vi "Begin.vi"(11 "Image Size":T1=enum."160x120") -> (0 "error out":errorcluster)   [LabVIEW 2013]
doc: "Called before other user functions, this VI is expected to open initial I/O refnums, load in file data, and do all program initialization. Notice that the <B>error out</B> terminal is simply used for data flow. Wiring it to other structures or subVIs ensures that this VI runs first."
uses:
  <vilib>/Rock Robotics/WPI/Camera/WPI_CameraImageSize.ctl
  <vilib>/Rock Robotics/SystemInterfaces/DIO/FPGA_DIOPWMChannel.ctl
  <vilib>/Rock Robotics/WPI/Solenoid/WPI_SolenoidChannel.ctl
  <vilib>/Rock Robotics/SystemInterfaces/Typedef/FPGA_TypedefDigitalModule.ctl
  <vilib>/Rock Robotics/SystemInterfaces/DIO/FPGA_DIOChannel.ctl
  <vilib>/Rock Robotics/SystemInterfaces/DIO/FPGA_DIORelayChannel.ctl
  <vilib>/Rock Robotics/WPI/DriverStation/WPI_DriverStationRobotMode2.ctl
  <vilib>/Rock Robotics/WPI/Joystick/WPI_JoystickDeviceEnum.ctl
  <vilib>/Rock Robotics/WPI/MotorControl/WPI_MotorControlOpen Talon.vi
  <vilib>/Rock Robotics/WPI/Solenoid/WPI_SolenoidOpenSingle.vi
  <vilib>/Rock Robotics/WPI/Compressor/WPI_CompressorGetSetRefNum.vi
  Robot Global Data.vi
  <vilib>/Rock Robotics/WPI/Camera/WPI_CameraWhite Balance Values.ctl
  <vilib>/Rock Robotics/WPI/Camera/WPI_CameraExposure Values.ctl
  <vilib>/Rock Robotics/WPI/Camera/WPI_CameraFrameRate.ctl
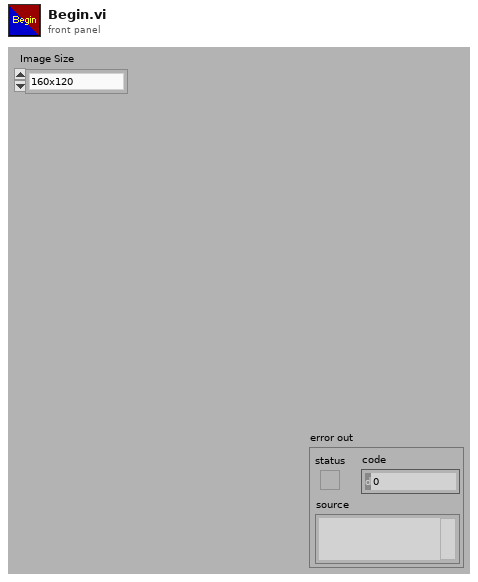
[diagram p1: front panel]
types:
  T1 = typedef "WPI_CameraImageSize.ctl" = enum16{"640x480", "320x240", "160x120"}
  T2 = typedef "FPGA_DIOPWMChannel.ctl" = enum8{"PWM 1", "PWM 2", "PWM 3", "PWM 4", "PWM 5", "PWM 6", "PWM 7", "PWM 8", "PWM 9", "PWM 10", "Invalid"}
  T3 = typedef "WPI_SolenoidChannel.ctl" = enum8{"Solenoid 1", "Solenoid 2", "Solenoid 3", "Solenoid 4", "Solenoid 5", "Solenoid 6", "Solenoid 7", "Solenoid 8", "Invalid"}
  T4 = typedef "FPGA_DIORelayChannel.ctl" = enum8{"Relay 1", "Relay 2", "Relay 3", "Relay 4", "Relay 5", "Relay 6", "Relay 7", "Relay 8", "Invalid"}
  T5 = typedef "FPGA_DIOChannel.ctl" = enum8{"DIO 1", "DIO 2", "DIO 3", "DIO 4", "DIO 5", "DIO 6", "DIO 7", "DIO 8", "DIO 9", "DIO 10", "DIO 11", "DIO 12", "DIO 13", "DIO 14", "Invalid"}
  T6 = typedef "WPI_JoystickDeviceEnum.ctl" = enum16{"USB 1", "USB 2", "USB 3", "USB 4", "Kinect 1", "Kinect 2"}
  T7 = typedef "WPI_DriverStationRobotMode2.ctl" = enum16{"Autonomous Disabled", "Autonomous Enabled", "Teleop Disabled", "Teleop Enabled", "Timeout", "Finish", "Test Disabled", "Test Enabled"}
  T8 = typedef "WPI_CameraFrameRate.ctl" = u32
  T9 = typedef "WPI_CameraExposure Values.ctl" = enum16{"Auto", "Flicker-free 50 Hz", "Flicker-free 60 Hz", "Hold current"}
  T10 = typedef "WPI_CameraWhite Balance Values.ctl" = enum16{"Auto", "Fixed indoor", "Fixed outdoor 1", "Fixed outdoor 2", "Fixed fluorescent 1", "Fixed fluorescent 2", "Hold current"}
  T11 = typedef "WPI_MotorControlDeviceRef.ctl" = cluster{"DeviceStatus":errorcluster, "Type":enum16{"PWM", "CAN"}, "PWM":cluster{"Digital Module":T12, "PWM Channel":T2, "DeadBand":T13}, "CAN":cluster{"Device Number":u8, "Control Mode":T14, "Semaphore":T15, "Max Vout":dbl}, "Invert":bool, "TransformRef":T16, "InvTransformRef":T16}
  T12 = typedef "FPGA_TypedefDigitalModule.ctl" = enum16{"Digital Module 1", "Digital Module 2"}
  T13 = typedef "WPI_PWMDeadband.ctl" = cluster{"Name":string, "maxPositivePwm":i32, "minPositivePwm":i32, "centerPwm":i32, "maxNegativePwm":i32, "minNegativePwm":i32, "angularRange":u16}
  T14 = typedef "WPI_CANJaguar_ControlMode.ctl" = enum8{"Percent VBus", "Current", "Speed", "Position", "Voltage"}
  T15 = typedef "Semaphore RefNum" = refnum<k1>
  T16 = typedef "WPI_PWMTransform_ConPane.ctl" = refnum<vi>
  T17 = typedef "WPI_SolenoidDevRef.ctl" = cluster{"DevStatus":errorcluster, "Solenoid Module":T18, "Forward Solenoid Channel":T3, "Reverse Solenoid Channel":T3}
  T18 = typedef "FPGA_TypedefSolenoidModule.ctl" = enum16{"Solenoid Module 1", "Solenoid Module 2"}
  T19 = typedef "WPI_CompressorDevRef.ctl" = cluster{"DevStatus":errorcluster, "DigitalInputDevRef":T20, "RelayDevRef":T21}
  T20 = typedef "WPI_DigitalInputDevRef.ctl" = cluster{"DevStatus":errorcluster, "DIO Channel":T5, "Digital Module":T12}
  T21 = typedef "WPI_RelayDevRef.ctl" = cluster{"DevStatus":errorcluster, "Relay Channel":T4, "Digital Module":T12, "Relay Direction":T22}
  T22 = typedef "WPI_RelayDirection.ctl" = enum16{"Both directions", "Forward only", "Reverse only"}
  T23 = typedef "WPI_CameraDevRef.ctl" = cluster{"Camera Address":string, "CameraStatus":errorcluster, "Acquire Image Notifier":refnum<notifier>}
  T24 = typedef "WPI_JoystickDevRef.ctl" = cluster{"Device":T6}
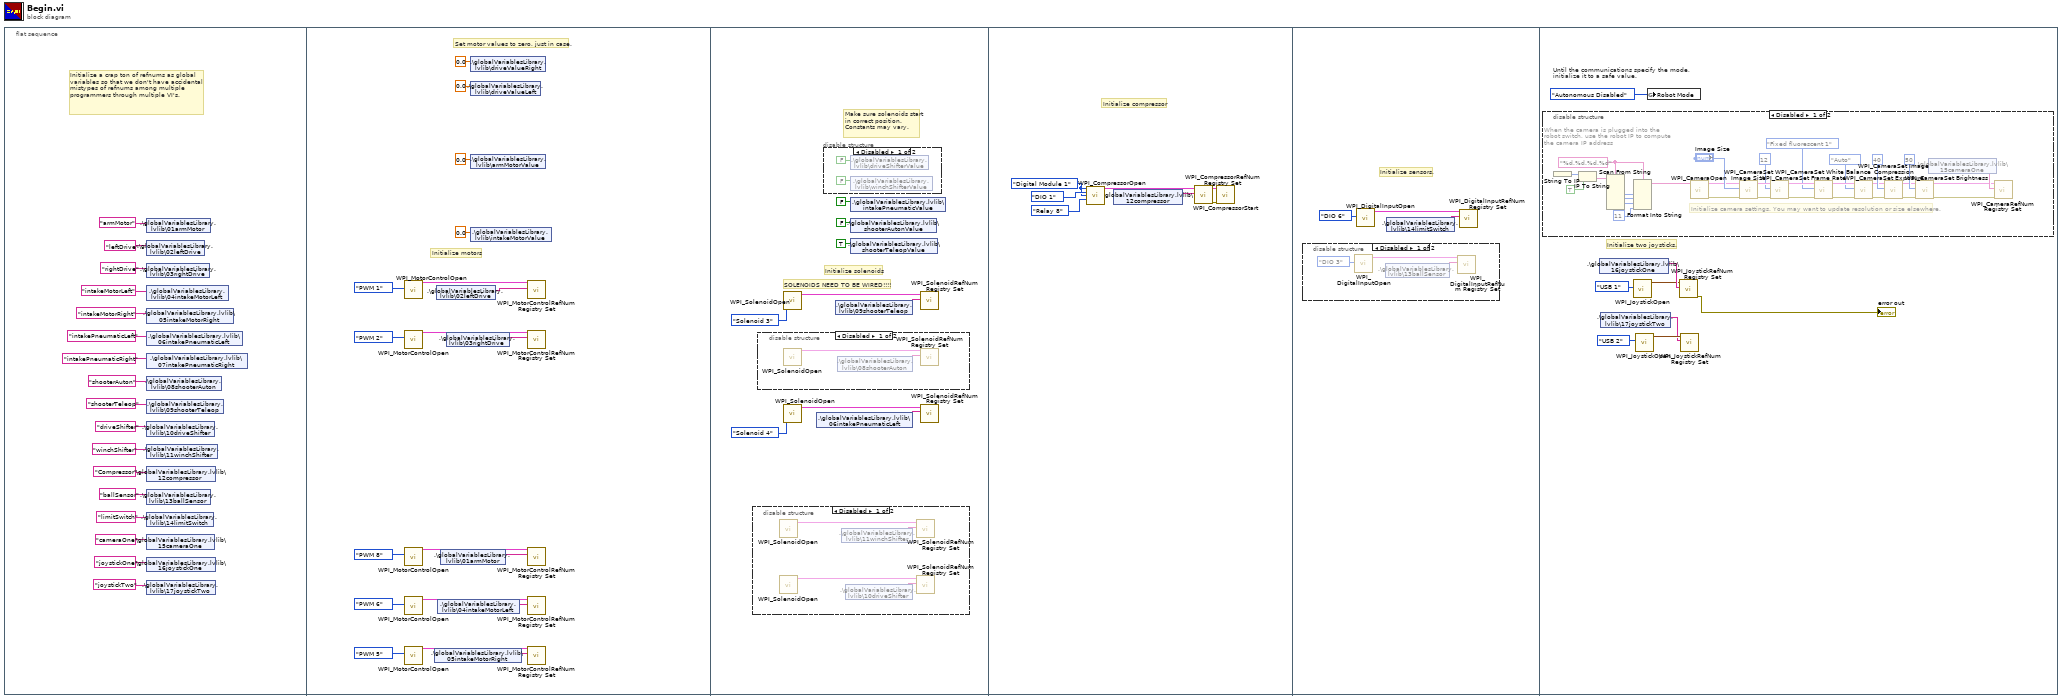
[diagram p0: block diagram]
diagram:
  n1 = flat-sequence {
    frame #0 {
      # "Initialize a crap ton of refnums as global variables so that we don't have accidental mistypes of refnums among multiple programmers through multiple VI's."
      n2 = shared-variable ".\\globalVariablesLibrary.lvlib\\01armMotor"("armMotor" ("armMotorRight")) -> ()  [unwired: 1 in, 1 out]
      n3 = shared-variable ".\\globalVariablesLibrary.lvlib\\02leftDrive"("leftDrive" ("backLeftMotor")) -> ()  [unwired: 1 in, 1 out]
      n4 = shared-variable ".\\globalVariablesLibrary.lvlib\\03rightDrive"("rightDrive" ("backRightMotor")) -> ()  [unwired: 1 in, 1 out]
      n5 = shared-variable ".\\globalVariablesLibrary.lvlib\\04intakeMotorLeft"("intakeMotorLeft" ("intakeMotorLeft")) -> ()  [unwired: 1 in, 1 out]
      n6 = shared-variable ".\\globalVariablesLibrary.lvlib\\05intakeMotorRight"("intakeMotorRight" ("intakeMotorRight")) -> ()  [unwired: 1 in, 1 out]
      n7 = shared-variable ".\\globalVariablesLibrary.lvlib\\06intakePneumaticLeft"("intakePneumaticLeft" ("intakePneumaticLeft")) -> ()  [unwired: 1 in, 1 out]
      n8 = shared-variable ".\\globalVariablesLibrary.lvlib\\07intakePneumaticRight"("intakePneumaticRight" ("intakePneumaticRight")) -> ()  [unwired: 1 in, 1 out]
      n9 = shared-variable ".\\globalVariablesLibrary.lvlib\\08shooterAuton"("shooterAuton" ("camerone")) -> ()  [unwired: 1 in, 1 out]
      n10 = shared-variable ".\\globalVariablesLibrary.lvlib\\09shooterTeleop"("shooterTeleop" ("camerone")) -> ()  [unwired: 1 in, 1 out]
      n11 = shared-variable ".\\globalVariablesLibrary.lvlib\\10driveShifter"("driveShifter" ("11driveShifter")) -> ()  [unwired: 1 in, 1 out]
      n12 = shared-variable ".\\globalVariablesLibrary.lvlib\\11winchShifter"("winchShifter" ("12winchShifter")) -> ()  [unwired: 1 in, 1 out]
      n13 = shared-variable ".\\globalVariablesLibrary.lvlib\\12compressor"("Compressor" ("compressor")) -> ()  [unwired: 1 in, 1 out]
      n14 = shared-variable ".\\globalVariablesLibrary.lvlib\\13ballSensor"("ballSensor" ("ballSensor")) -> ()  [unwired: 1 in, 1 out]
      n15 = shared-variable ".\\globalVariablesLibrary.lvlib\\14limitSwitch"("limitSwitch" ("limitSwitch")) -> ()  [unwired: 1 in, 1 out]
      n16 = shared-variable ".\\globalVariablesLibrary.lvlib\\15cameraOne"("cameraOne" ("camerone")) -> ()  [unwired: 1 in, 1 out]
      n17 = shared-variable ".\\globalVariablesLibrary.lvlib\\16joystickOne"("joystickOne" ("joystickOne")) -> ()  [unwired: 1 in, 1 out]
      n18 = shared-variable ".\\globalVariablesLibrary.lvlib\\17joystickTwo"("joystickTwo" ("joystickTwo")) -> ()  [unwired: 1 in, 1 out]
    }
    frame #1 {
      # "Set motor values to zero, just in case."
      # "Initialize motors"
      n19 = call-poly <vilib>:"WPI_MotorControlOpen.vi"("PWM Channel"=FPGA_DIOPWMChannel."PWM 1") -> ("MotorControlDeviceRef"=w36:T11)  [unwired: 9 in, 1 out]
      n20 = call-poly <vilib>:"WPI_MotorControlOpen.vi"("PWM Channel"=FPGA_DIOPWMChannel."PWM 2") -> ("MotorControlDeviceRef"=w35:T11)  [unwired: 9 in, 1 out]
      n21 = call-poly <vilib>:"WPI_MotorControlOpen.vi"("PWM Channel"=FPGA_DIOPWMChannel."PWM 8") -> ("MotorControlDeviceRef"=w27:T11)  [unwired: 9 in, 1 out]
      n22 = call-poly <vilib>:"WPI_MotorControlOpen.vi"("PWM Channel"=FPGA_DIOPWMChannel."PWM 6") -> ("MotorControlDeviceRef"=w21:T11)  [unwired: 9 in, 1 out]
      n23 = call-poly <vilib>:"WPI_MotorControlOpen.vi"("PWM Channel"=FPGA_DIOPWMChannel."PWM 5") -> ("MotorControlDeviceRef"=w22:T11)  [unwired: 9 in, 1 out]
      n24 = shared-variable ".\\globalVariablesLibrary.lvlib\\05intakeMotorRight"() -> (w23:string)  [unwired: 1 in, 1 out]
      n25 = shared-variable ".\\globalVariablesLibrary.lvlib\\02leftDrive"() -> (w18:string)  [unwired: 1 in, 1 out]
      n26 = shared-variable ".\\globalVariablesLibrary.lvlib\\04intakeMotorLeft"() -> (w20:string)  [unwired: 1 in, 1 out]
      n27 = shared-variable ".\\globalVariablesLibrary.lvlib\\01armMotor"() -> (w26:string)  [unwired: 1 in, 1 out]
      n28 = shared-variable ".\\globalVariablesLibrary.lvlib\\03rightDrive"() -> (w34:string)  [unwired: 1 in, 1 out]
      n29 = shared-variable ".\\globalVariablesLibrary.lvlib\\driveValueRight"(0.0 ("driveValueFrontRight")) -> ()  [unwired: 1 in, 1 out]
      n30 = shared-variable ".\\globalVariablesLibrary.lvlib\\driveValueLeft"(0.0 ("driveValueFrontLeft")) -> ()  [unwired: 1 in, 1 out]
      n31 = shared-variable ".\\globalVariablesLibrary.lvlib\\armMotorValue"(0.0 ("armMotorValueLeft")) -> ()  [unwired: 1 in, 1 out]
      n32 = shared-variable ".\\globalVariablesLibrary.lvlib\\intakeMotorValue"(0.0 ("intakeMotorValueLeft")) -> ()  [unwired: 1 in, 1 out]
      n33 = call <vilib>:"WPI_MotorControlRefNum Registry Set.vi"("refnum name"=w18, "MotorControlDevRef"=w36) -> ()  [unwired: 8 in, 2 out]
      n34 = call <vilib>:"WPI_MotorControlRefNum Registry Set.vi"("refnum name"=w34, "MotorControlDevRef"=w35) -> ()  [unwired: 8 in, 2 out]
      n35 = call <vilib>:"WPI_MotorControlRefNum Registry Set.vi"("refnum name"=w26, "MotorControlDevRef"=w27) -> ()  [unwired: 8 in, 2 out]
      n36 = call <vilib>:"WPI_MotorControlRefNum Registry Set.vi"("refnum name"=w20, "MotorControlDevRef"=w21) -> ()  [unwired: 8 in, 2 out]
      n37 = call <vilib>:"WPI_MotorControlRefNum Registry Set.vi"("refnum name"=w23, "MotorControlDevRef"=w22) -> ()  [unwired: 8 in, 2 out]
    }
    frame #2 {
      # "SOLENOIDS NEED TO BE WIRED!!!!"
      # "Initialize solenoids"
      # "Make sure solenoids start in correct position. Constants may vary."
      n38 = disable-structure shown="Disabled" {
        frame Disabled {
          n39 = call-poly <vilib>:"WPI_SolenoidOpen.vi"() -> ("SolenoidDevRef"=w49:T17)  [unwired: 10 in, 1 out]
          n40 = call-poly <vilib>:"WPI_SolenoidOpen.vi"() -> ("SolenoidDevRef"=w50:T17)  [unwired: 10 in, 1 out]
          n41 = shared-variable ".\\globalVariablesLibrary.lvlib\\11winchShifter"() -> (w48:string)  [unwired: 1 in, 1 out]
          n42 = shared-variable ".\\globalVariablesLibrary.lvlib\\10driveShifter"() -> (w51:string)  [unwired: 1 in, 1 out]
          n43 = call <vilib>:"WPI_SolenoidRefNum Registry Set.vi"("refnum name"=w48, "SolenoidDevRef"=w49) -> ()  [unwired: 8 in, 2 out]
          n44 = call <vilib>:"WPI_SolenoidRefNum Registry Set.vi"("refnum name"=w51, "SolenoidDevRef"=w50) -> ()  [unwired: 8 in, 2 out]
        }
        frame Enabled {
        }
      }
      n45 = disable-structure shown="Disabled" {
        frame Disabled {
          n46 = call-poly <vilib>:"WPI_SolenoidOpen.vi"() -> ("SolenoidDevRef"=w47:T17)  [unwired: 10 in, 1 out]
          n47 = shared-variable ".\\globalVariablesLibrary.lvlib\\08shooterAuton"() -> (w46:string)  [unwired: 1 in, 1 out]
          n48 = call <vilib>:"WPI_SolenoidRefNum Registry Set.vi"("refnum name"=w46, "SolenoidDevRef"=w47) -> ()  [unwired: 8 in, 2 out]
        }
        frame Enabled {
        }
      }
      n49 = call-poly <vilib>:"WPI_SolenoidOpen.vi"("Solenoid Channel"=WPI_SolenoidChannel."Solenoid 3") -> ("SolenoidDevRef"=w41:T17)  [unwired: 9 in, 1 out]
      n50 = call-poly <vilib>:"WPI_SolenoidOpen.vi"("Solenoid Channel"=WPI_SolenoidChannel."Solenoid 4") -> ("SolenoidDevRef"=w43:T17)  [unwired: 9 in, 1 out]
      n51 = shared-variable ".\\globalVariablesLibrary.lvlib\\06intakePneumaticLeft"() -> (w44:string)  [unwired: 1 in, 1 out]
      n52 = disable-structure shown="Disabled" {
        frame Disabled {
          n53 = shared-variable ".\\globalVariablesLibrary.lvlib\\driveShifterValue"(FALSE ("driveShifterValue")) -> ()  [unwired: 1 in, 1 out]
          n54 = shared-variable ".\\globalVariablesLibrary.lvlib\\winchShifterValue"(FALSE ("winchShifterValue")) -> ()  [unwired: 1 in, 1 out]
        }
        frame Enabled {
        }
      }
      n55 = shared-variable ".\\globalVariablesLibrary.lvlib\\09shooterTeleop"() -> (w40:string)  [unwired: 1 in, 1 out]
      n56 = shared-variable ".\\globalVariablesLibrary.lvlib\\intakePneumaticValue"(FALSE ("shotTypeValue")) -> ()  [unwired: 1 in, 1 out]
      n57 = shared-variable ".\\globalVariablesLibrary.lvlib\\shooterAutonValue"(FALSE ("shotTypeValue")) -> ()  [unwired: 1 in, 1 out]
      n58 = shared-variable ".\\globalVariablesLibrary.lvlib\\shooterTeleopValue"(TRUE ("shooterValue")) -> ()  [unwired: 1 in, 1 out]
      n59 = call <vilib>:"WPI_SolenoidRefNum Registry Set.vi"("refnum name"=w40, "SolenoidDevRef"=w41) -> ()  [unwired: 8 in, 2 out]
      n60 = call <vilib>:"WPI_SolenoidRefNum Registry Set.vi"("refnum name"=w44, "SolenoidDevRef"=w43) -> ()  [unwired: 8 in, 2 out]
    }
    frame #3 {
      w55 = FPGA_TypedefDigitalModule."Digital Module 1" ("Pressure Switch Digital Module (Module 1)")
      # "Initialize compressor"
      n61 = call <vilib>:"WPI_CompressorOpen.vi"("Pressure Switch Digital Module (Module 1)"=w55, "Pressure Switch DIO Channel"=FPGA_DIOChannel."DIO 1", "Relay Digital Module (Module 1)"=w55, "Relay Channel"=FPGA_DIORelayChannel."Relay 8") -> ("CompressorDevRef"=w60:T19)  [unwired: 10 in, 1 out]
      n62 = shared-variable ".\\globalVariablesLibrary.lvlib\\12compressor"() -> (w57:string)  [unwired: 1 in, 1 out]
      n63 = call <vilib>:"WPI_CompressorRefNum Registry Set.vi"("refnum name"=w57, "CompressorDevRef"=w60) -> ("error out"=w59:errorcluster, "CompressorDevRef"=w58:T19)  [unwired: 8 in]
      n64 = call <vilib>:"WPI_CompressorStart.vi"("error in (no error)"=w59, "CompressorDevRef"=w58) -> ()  [unwired: 8 in, 2 out]
    }
    frame #4 {
      # "Initialize sensors."
      n65 = disable-structure shown="Disabled" {
        frame Disabled {
          n66 = call <vilib>:"WPI_DigitalInputOpen.vi"("DIO Channel"=FPGA_DIOChannel."DIO 3") -> ("DigitalInputDevRef"=w65:T20)  [unwired: 9 in, 1 out]
          n67 = shared-variable ".\\globalVariablesLibrary.lvlib\\13ballSensor"() -> (w66:string)  [unwired: 1 in, 1 out]
          n68 = call <vilib>:"WPI_DigitalInputRefNum Registry Set.vi"("refnum name"=w66, "DigitalInputDevRef"=w65) -> ()  [unwired: 8 in, 2 out]
        }
        frame Enabled {
        }
      }
      n69 = call <vilib>:"WPI_DigitalInputOpen.vi"("DIO Channel"=FPGA_DIOChannel."DIO 6") -> ("DigitalInputDevRef"=w62:T20)  [unwired: 9 in, 1 out]
      n70 = shared-variable ".\\globalVariablesLibrary.lvlib\\14limitSwitch"() -> (w61:string)  [unwired: 1 in, 1 out]
      n71 = call <vilib>:"WPI_DigitalInputRefNum Registry Set.vi"("refnum name"=w61, "DigitalInputDevRef"=w62) -> ()  [unwired: 8 in, 2 out]
    }
    frame #5 {
      # "Initialize two joysticks."
      # "Until the communications specify the mode,\ninitialize it to a safe value."
      n72 = disable-structure shown="Disabled" {
        frame Disabled {
          w77 = "%d.%d.%d.%d" ("format string")
          # "When the camera is plugged into the\nrobot switch, use the robot IP to compute\nthe camera IP address"
          # "Initialize camera settings. You may want to update resolution or size elsewhere."
          n73 = String To IP() -> (0:w83:u32)  [unwired: 1 in]
          n74 = IP To String(1:TRUE ("dot notation? (F)"), 2:w83) -> (0:w81:string)
          n75 = Scan From String(format string=w77, input string=w81) -> (output 1=w80:i32, output 2=w79:i32, output 3=w78:i32)  [unwired: 7 in, 3 out]
          n76 = Format Into String(format string=w77, w80, w79, w78, 11 ("Compression")) -> (resulting string=w76:string)  [unwired: 2 in, 1 out]
          n77 = call <vilib>:"WPI_CameraOpen.vi"("Camera Address"=w76) -> ("error out"=w94:errorcluster, "CameraDevRef"=w95:T23)  [unwired: 1 in, 8 out]
          n78 = call <vilib>:"WPI_CameraSet Image Size.vi"("error in (no error)"=w94, "Image Size"="Image Size", "CameraDevRef"=w95) -> ("error out"=w93:errorcluster, "CameraDevRef Out"=w96:T23)  [unwired: 7 out]
          n79 = call <vilib>:"WPI_CameraSet Frame Rate.vi"("error in (no error)"=w93, "Frame Rate (fps)"=T8 12, "CameraDevRef"=w96) -> ("error out"=w92:errorcluster, "CameraDevRef Out"=w98:T23)  [unwired: 7 out]
          n80 = call <vilib>:"WPI_CameraSet White Balance.vi"("error in (no error)"=w92, "White Balance"=WPI_CameraWhite_Balance_Values."Fixed fluorescent 1", "CameraDevRef"=w98) -> ("error out"=w91:errorcluster, "CameraDevRef Out"=w97:T23)  [unwired: 7 out]
          n81 = call <vilib>:"WPI_CameraSet Exposure.vi"("error in (no error)"=w91, "Exposure"=WPI_CameraExposure_Values."Auto", "CameraDevRef"=w97) -> ("error out"=w90:errorcluster, "CameraDevRef Out"=w100:T23)  [unwired: 7 out]
          n82 = call <vilib>:"WPI_CameraSet Image Compression.vi"("error in (no error)"=w90, "Compression"=40, "CameraDevRef"=w100) -> ("error out"=w89:errorcluster, "CameraDevRef Out"=w99:T23)  [unwired: 7 out]
          n83 = call <vilib>:"WPI_CameraSet Brightness.vi"("error in (no error)"=w89, "Brightness"=50, "CameraDevRef"=w99) -> ("error out"=w87:errorcluster, "CameraDevRef Out"=w88:T23)  [unwired: 7 out]
          n84 = shared-variable ".\\globalVariablesLibrary.lvlib\\15cameraOne"() -> (w104:string)  [unwired: 1 in, 1 out]
          n85 = call <vilib>:"WPI_CameraRefNum Registry Set.vi"("error in (no error)"=w87, "refnum name"=w104, "CameraDevRef"=w88) -> ()  [unwired: 9 out]
        }
        frame Enabled {
        }
      }
      n86 = shared-variable ".\\globalVariablesLibrary.lvlib\\16joystickOne"() -> (w73:string)  [unwired: 1 in, 1 out]
      n87 = shared-variable ".\\globalVariablesLibrary.lvlib\\17joystickTwo"() -> (w68:string)  [unwired: 1 in, 1 out]
      n88 = call <vilib>:"WPI_JoystickOpen.vi"("JoystickDevice"=WPI_JoystickDeviceEnum."USB 1") -> ("JoystickDevRef"=w72:T24)  [unwired: 10 in]
      n89 = call <vilib>:"WPI_JoystickOpen.vi"("JoystickDevice"=WPI_JoystickDeviceEnum."USB 2") -> ("JoystickDevRef"=w69:T24)  [unwired: 10 in]
      n90 = global write "Robot Global Data.vi" "Robot Mode"(WPI_DriverStationRobotMode2."Autonomous Disabled" ("Robot Mode")) -> ()
      n91 = call <vilib>:"WPI_JoystickRefNum Registry Set.vi"("refnum name"=w73, "JoystickDevRef"=w72) -> ("error out"=→"error out":errorcluster)  [unwired: 8 in, 1 out]
      n92 = call <vilib>:"WPI_JoystickRefNum Registry Set.vi"("refnum name"=w68, "JoystickDevRef"=w69) -> ()  [unwired: 8 in, 2 out]
    }
  }
